vi "Framework Test.vi"() -> ()   [LabVIEW 2017]
uses:
  Source/Shared/Typedefs/DSF.Shared.Typedefs.Data Type.ctl
  Source/Shared/Typedefs/DSF.Shared.Typedefs.Direction.ctl
  Source/Shared/Typedefs/DSF.Shared.Typedefs.Cycle Timing Factors.ctl
  Source/Plugins/Reflective Memory/DSF.Transceiver.GE Reflective Memory.lvclass
  Source/Plugins/PXImc/DSF.Transceiver.PXImc.lvclass
  Source/Plugins/UDP/DSF.Transceiver.UDP.lvclass
  Source/Engine/Classes/Framework/DSF.Engine.Framework.lvclass
  <vilib>/Platform/TimedLoop/XDataNode/timing_clust.ctl
  <vilib>/Platform/TimedLoop/XDataNode/nitl_modes.ctl
  <vilib>/Platform/TimedLoop/XDataNode/wakeup.ctl
  <vilib>/National Instruments/Memory Manager/Classes/Pointer/Memory.Pointer.lvclass/Memory.Pointer.ctl
  Source/Engine/Classes/Framework/DSF.Engine.Framework.lvclass/DSF.Engine.Framework.ctl
  Source/Engine/Classes/Plugin/DSF.Engine.Plugin.lvclass/DSF.Engine.Plugin.ctl
  Source/Engine/Classes/Timing/DSF.Engine.Timing.lvclass/DSF.Engine.Timing.ctl
  <vilib>/National Instruments/Memory Manager/Classes/Pointer/Memory.Pointer.New.4B.vi
  <vilib>/National Instruments/Memory Manager/Classes/Pointer/Memory.Pointer.Write.0D.U32.vi
  <vilib>/National Instruments/Memory Manager/Classes/Pointer/Memory.Pointer.New.1B.vi
  <vilib>/National Instruments/Memory Manager/Classes/Pointer/Memory.Pointer.Write.0D.Bool.vi
  <vilib>/National Instruments/Memory Manager/Classes/Pointer/Memory.Pointer.Read.0D.Bool.vi
  <vilib>/National Instruments/Memory Manager/Classes/Pointer/Memory.Pointer.Read.0D.I32.vi
  <vilib>/National Instruments/Memory Manager/Classes/Pointer/Memory.Pointer.Read.0D.U32.vi
  <vilib>/National Instruments/Memory Manager/Classes/Pointer/Memory.Pointer.Write.0D.I32.vi
  <vilib>/National Instruments/Memory Manager/Classes/Pointer/Memory.Pointer.Allocate.vi
  <vilib>/National Instruments/Memory Manager/Classes/Pointer/Memory.Pointer.Write.No Check.0D.U32.vi
  <vilib>/National Instruments/Memory Manager/Classes/Pointer/Memory.Pointer.Parameter Check.Null Pointer.vi
  <vilib>/National Instruments/Memory Manager/Classes/Pointer/Memory.Pointer.Parameter Check.Subset.vi
  <vilib>/National Instruments/Memory Manager/Classes/Pointer/Memory.Pointer.Write.No Check.0D.Bool.vi
  <vilib>/National Instruments/Memory Manager/Classes/Pointer/Memory.Pointer.Read.No Check.0D.Bool.vi
  <vilib>/National Instruments/Memory Manager/Classes/Pointer/Memory.Pointer.Read.No Check.0D.I32.vi
  <vilib>/National Instruments/Memory Manager/Classes/Pointer/Memory.Pointer.Read.No Check.0D.U32.vi
  <vilib>/National Instruments/Memory Manager/Classes/Pointer/Memory.Pointer.Write.No Check.0D.I32.vi
  Source/Engine/Classes/Framework/DSF.Engine.Framework.Set Iteration.vi
  Source/Engine/Classes/Framework/DSF.Engine.Framework.Tx.Async.vi
  Source/Engine/Classes/Framework/DSF.Engine.Framework.Get State.vi
  Source/Engine/Classes/State/DSF.Engine.State.Framework.Get Active Plugins.vi
  Source/Engine/Classes/Framework/DSF.Engine.Framework.Get Iteration.vi
  Source/Engine/Classes/Plugin/DSF.Engine.Plugin.Iteration.Increment.vi
  Source/Engine/Classes/Plugin/DSF.Engine.Plugin.Is Active.vi
  <vilib>/National Instruments/Memory Manager/Classes/Pointer/Memory.Pointer.Set Address.vi
  <vilib>/National Instruments/Memory Manager/Classes/Pointer/Memory.Pointer.Set Size.vi
  <vilib>/National Instruments/Memory Manager/Classes/Pointer/Memory.Pointer.Set Allocated.vi
  <vilib>/National Instruments/Memory Manager/Classes/Pointer/Memory.Pointer.Get Address.vi
  <vilib>/National Instruments/Memory Manager/Classes/Pointer/Memory.Pointer.Errors.vi
  <vilib>/National Instruments/Memory Manager/Classes/Pointer/Memory.Pointer.Errors.Null Pointer.vi
  <vilib>/National Instruments/Memory Manager/Classes/Pointer/Memory.Pointer.Errors.Out of Bounds.vi
  <vilib>/National Instruments/Memory Manager/Classes/Pointer/Memory.Pointer.Get Size.vi
  Source/Engine/Classes/Plugin/DSF.Engine.Plugin.Get Timing.vi
  Source/Engine/Classes/Timing/DSF.Engine.Timing.Iteration.Increment.vi
  Source/Engine/Classes/Plugin/DSF.Engine.Plugin.Set Timing.vi
  Source/Engine/Classes/Timing/DSF.Engine.Timing.Is Active Cycle.vi
  <vilib>/National Instruments/Memory Manager/Classes/Pointer/Memory.Pointer.Errors.Create Error.vi
  <vilib>/NI/Static Error Handling/VIs/Static Error Handling.Source Buffer.Write.String.vi
  <vilib>/National Instruments/Memory Manager/Classes/Pointer/Memory.Pointer.Errors.Write Pointer Size.vi
  <vilib>/NI/Static Error Handling/VIs/Static Error Handling.Source Buffer.Write.Numeric.Scalar.Base10.vi
  <vilib>/NI/Static Error Handling/VIs/Static Error Handling.Source Buffer.Write.Numeric.Scalar.Base10 (U64).vi
  Source/Engine/Classes/Timing/DSF.Engine.Timing.Get Iteration.vi
  Source/Engine/Classes/Timing/DSF.Engine.Timing.Set Iteration.vi
  Source/Engine/Classes/Timing/DSF.Engine.Timing.Get Decimation.vi
  Source/Engine/Classes/Timing/DSF.Engine.Timing.Get Offset.vi
  <vilib>/NI/Static Error Handling/VIs/Static Error Handling.Error Cluster Constant.vi
  <vilib>/NI/Static Error Handling/VIs/Static Error Handling.Error Cluster Constant (512B).vi
  <vilib>/NI/Static Error Handling/VIs/Static Error Handling.Parameters.Status.Set.vi
  <vilib>/NI/Static Error Handling/VIs/Static Error Handling.Parameters.Code.Set.vi
  <vilib>/NI/Static Error Handling/VIs/Static Error Handling.Parameters.VI Source.Set.vi
  <vilib>/National Instruments/Memory Manager/Constants/Memory.Constants.vi
  <vilib>/National Instruments/Memory Manager/Constants/Memory.Constants.Library Name.vi
  <vilib>/National Instruments/Memory Manager/Classes/Pointer/Memory.Pointer.Errors.Get Info.vi
  Source/Engine/Classes/Plugin/DSF.Engine.Plugin.Tx.Async.vi
  <vilib>/National Instruments/Memory Manager/Classes/Pointer/Memory.Pointer.lvclass
  <vilib>/platform/TimedLoop/XDataNode/XDataNode.xnode
  <vilib>/Platform/TimedLoop/XDataNode/XDNodeRunTimeDep.lvlib
  Source/Shared/Classes/Framework/DSF.Shared.Configuration.Framework.lvclass
  Source/Engine/Classes/Pointer/DSF.Engine.Pointer.DBL.lvclass
  Source/DSF.Shared.lvlib
panel:
  out "Framework duration":u32 format="%d us"
  out "Framework Error":errorcluster
  out "Tx duration":u32 format="%d us"
  out "Rx duration":u32 format="%d us"
  out "Actual PCL Frequency":dbl format="%.0pHz"
  out "UDP Rx 2 count":i32
  out "UDP Rx 1 count":i32
  out "UDP Rx 2":errorcluster
  out "UDP Rx 1":errorcluster
  out "UDP Rx 2 port":u16
  out "UDP Rx 2 bytes":i32
  out "UDP Rx 1 bytes":i32
  out "UDP Rx 1 port":u16
  in  "Transceiver Count":i32=1
  in  "Plugins":T4(array[cluster])=[{"plugin class"="udp", "channel count per transfer"=100, "transfer configs per group"=[{"random types?"=FALSE, "non-random type"=enum."DBL"}], "group configs"=[{"direction"=enum."Tx", "timing"={"Priority"=100, "Decimation"=1, "Offset"=0}}], "plugin timing"={"Priority"=100, "Decimation"=1, "Offset"=0}}]
  in  "Configuration Path":path=path "C:/Users/Admin/Desktop/test.json"
  out "Framework Iteration":i32 format="%d cycles"
  out "Actual Period":u32 format="%d us"
  in  "Target PCL Frequency":dbl=100.0 caption="Target Period" format="%.0pHz"
  in  "stop":bool
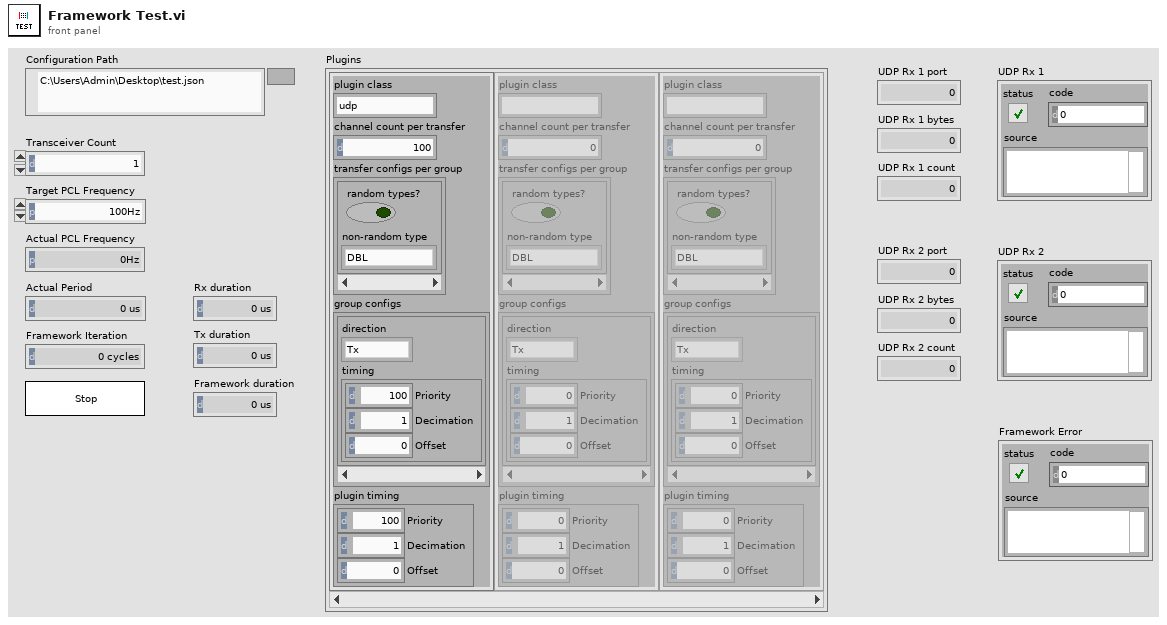
[diagram p1: front panel]
types:
  T1 = typedef "DSF.Shared.lvlib/DSF.Shared.Typedefs.Data Type.ctl" = enum8{"Bool", "SGL", "DBL", "I8", "I16", "I32", "I64", "U8", "U16", "U32", "U64"}
  T2 = typedef "DSF.Shared.lvlib/DSF.Shared.Typedefs.Direction.ctl" = enum8{"Tx", "Rx"}
  T3 = typedef "DSF.Shared.lvlib/DSF.Shared.Typedefs.Cycle Timing Factors.ctl" = cluster{"Priority":u64, "Decimation":u64, "Offset":u64}
  T4 = cluster{"plugin class":string, "channel count per transfer":i32, "transfer configs per group":cluster{"random types?":bool, "non-random type":T1}[], "group configs":cluster{"direction":T2, "timing":T3}[], "plugin timing":T3}[]
  T5 = typedef "DSF.Shared.lvlib/DSF.Shared.Refactor.Typedefs.Framework Configuration.Aggregate.ctl" = cluster{"Plugins":T6[]}
  T6 = typedef "DSF.Shared.lvlib/DSF.Shared.Refactor.Typedefs.Plugin Configuration.Aggregate.ctl" = cluster{"name":string, "class":string, "cycle timing":T3, "Transfer Groups":T7[]}
  T7 = typedef "DSF.Shared.lvlib/DSF.Shared.Refactor.Typedefs.Transfer Group Configuration.Aggregate.ctl" = cluster{"name":string, "direction":T2, "cycle timing":T3, "Transfers":T8[]}
  T8 = typedef "DSF.Shared.lvlib/DSF.Shared.Refactor.Typedefs.Transfer Configuration.ctl" = cluster{"name":string, "byte order":T9, "channel configurations":T10[]}
  T9 = typedef "DSF.Shared.lvlib/DSF.Shared.Typedefs.Byte Order.ctl" = enum8{"big-endian", "little-endian"}
  T10 = typedef "DSF.Shared.lvlib/DSF.Shared.Refactor.Typedefs.Channel Array Configuration.ctl" = cluster{"name":string, "data type":T1, "count":u64, "buffer offset":u64, "engine offset":u64}
  T11 = typedef "XDNodeRunTimeDep.lvlib/timing_clust.ctl" = cluster{"Expected End [f-1]":u64, "Actual End [f-1]":u64, "Finished Late? [f-1]":bool, "Expected End [i-1]":u64, "Actual End [i-1]":u64, "Finished Late? [i-1]":bool, "Expected Start [i]":u64, "Actual Start [i]":u64, "Expected Start [f]":u64, "Actual Start [f]":u64, "Source Name":string, "Structure Name":string, "Period":i64, "Deadline":i64, "Offset":i64, "Start":i64, "Priority":i32, "Timeout":i32, "Mode":T12, "Wakeup Reason":T13, "Error":errorcluster, "Source Type":string, "Secondary Source Type":string, "Global End Time":u64, "Global Start Time":u64, "Frame Duration":u64, "Iteration Duration":u64, "Assigned CPU":i32, "I/O Scan Engine Mode":u32}
  T12 = typedef "XDNodeRunTimeDep.lvlib/nitl_modes.ctl" = enum32{"No Change", "Process missed periods, maintain original phase", "Discard missed periods, maintain original phase", "Process missed periods, ignore original phase", "Discard missed periods, ignore original phase"}
  T13 = typedef "XDNodeRunTimeDep.lvlib/wakeup.ctl" = enum32{"Normal", "Aborted", "Asynchronous wakeup", "Timing source error", "Timed loop error", "Timeout"}
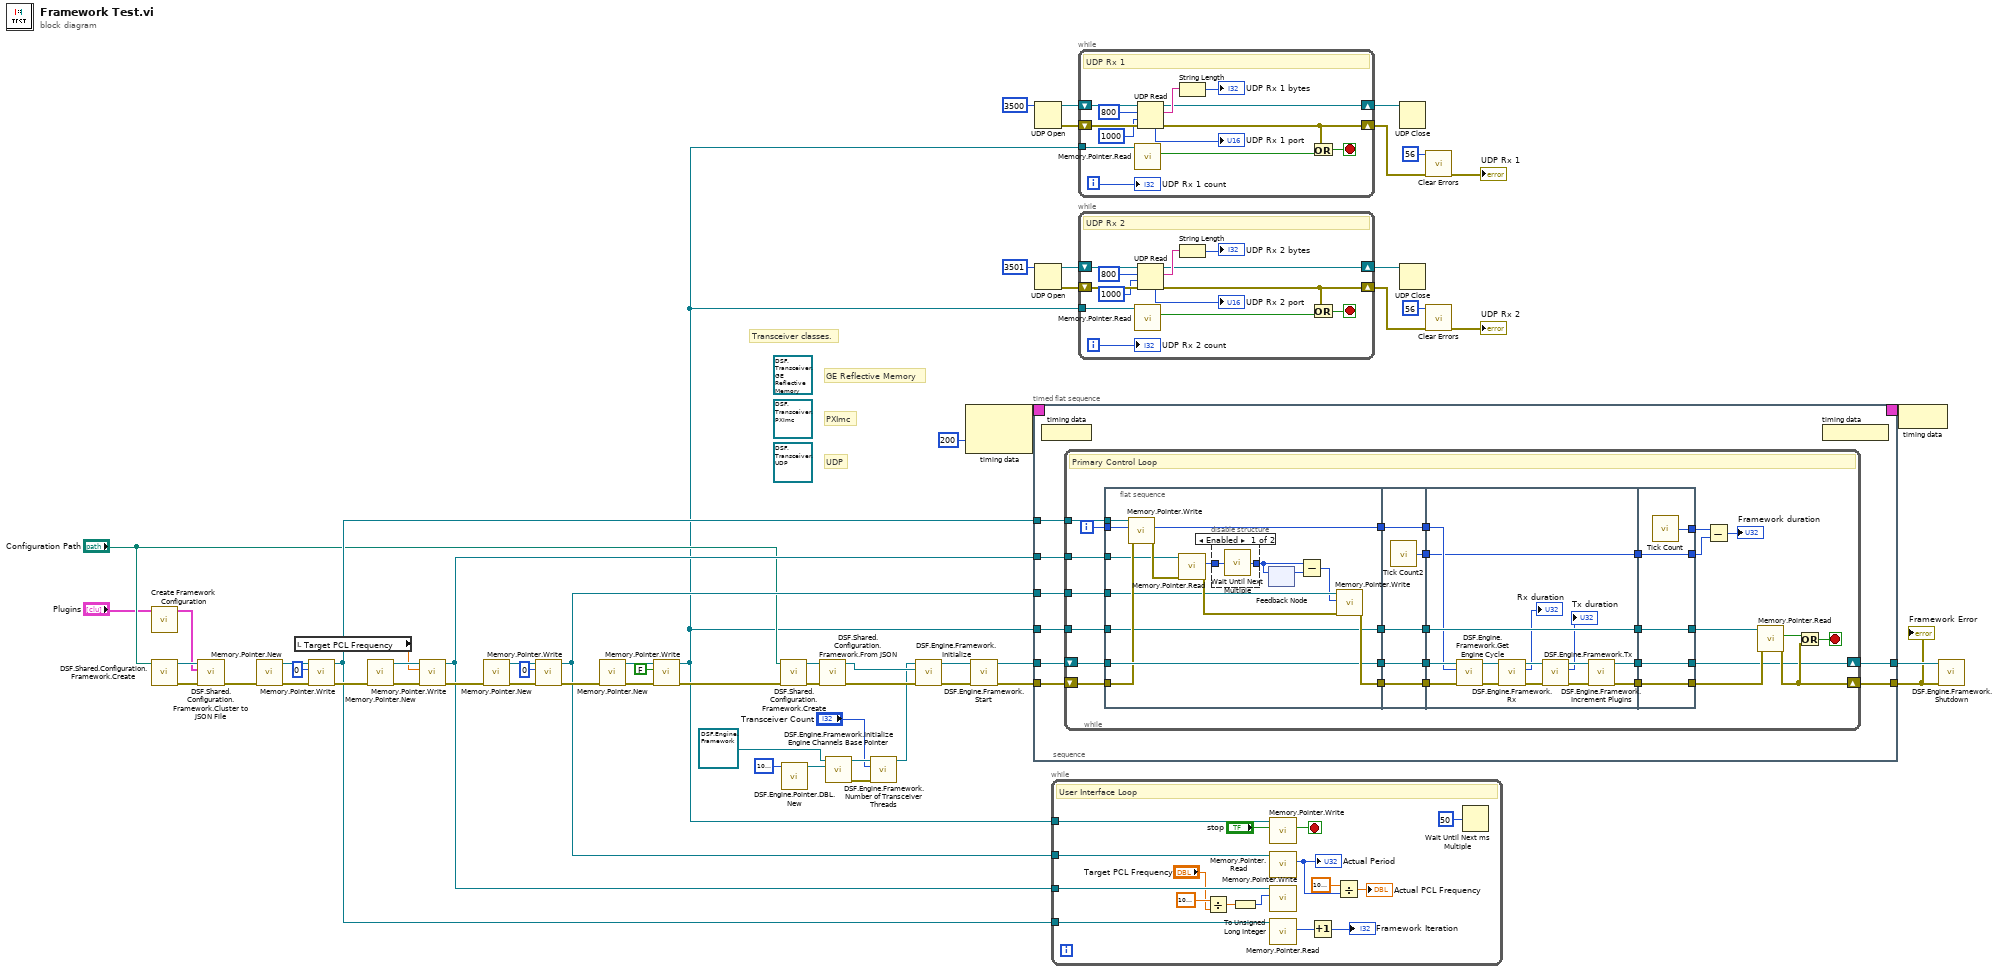
[diagram p0: block diagram]
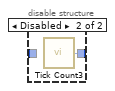
[diagram p2: hidden frame]
diagram:
  (unwired) refnum<class "DSF.Transceiver.UDP.lvclass"> refnum ("DSF UDP Transceiver")
  (unwired) refnum<class "DSF.Transceiver.PXImc.lvclass"> refnum ("DSF PXImc Transceiver")
  (unwired) refnum<class "DSF.Transceiver.GE Reflective Memory.lvclass"> refnum ("DSF GE Reflective Memory Transceiver")
  # "Transceiver classes."
  # "UDP"
  # "PXImc"
  # "GE Reflective Memory"
  n1 = call "Create Framework Configuration.vi"("Plugins"="Plugins") -> ("Framework Configuration"=w28:T5)  [unwired: 10 in]
  n2 = call "DSF.Shared.Configuration.Framework.Create.vi"("configuration path"="Configuration Path") -> ("error out"=w29:errorcluster, "Framework Configuration"=w30:refnum<class "DSF.Shared.Configuration.Framework.lvclass">)  [unwired: 9 in]
  n3 = call "DSF.Shared.Configuration.Framework.Cluster to JSON File.vi"("error in (no error)"=w29, "Framework Configuration"=w28, "Framework Configuration in"=w30) -> ("error out"=w27:errorcluster)  [unwired: 7 in, 1 out]
  n4 = call-poly <vilib>:"Memory.Pointer.New.vi"("error in (no error)"=w27) -> ("error out"=w37:errorcluster, "Pointer"=w39:refnum<class "Memory.Pointer.lvclass">)  [unwired: 9 in]
  n5 = local read "Target PCL Frequency"() -> (w47:dbl)
  n6 = call-poly <vilib>:"Memory.Pointer.Write.vi"("error in (no error)"=w37, "value"=u32 0, "Pointer in"=w39) -> ("error out"=w36:errorcluster, "Pointer out"=w33:refnum<class "Memory.Pointer.lvclass">)  [unwired: 5 in, 2 out]
  n7 = call-poly <vilib>:"Memory.Pointer.New.vi"("error in (no error)"=w36) -> ("error out"=w46:errorcluster, "Pointer"=w48:refnum<class "Memory.Pointer.lvclass">)  [unwired: 9 in]
  n8 = call-poly <vilib>:"Memory.Pointer.Write.vi"("error in (no error)"=w46, "value"=w47, "Pointer in"=w48) -> ("error out"=w45:errorcluster, "Pointer out"=w40:refnum<class "Memory.Pointer.lvclass">)  [unwired: 5 in, 2 out]
  n9 = call-poly <vilib>:"Memory.Pointer.New.vi"("error in (no error)"=w45) -> ("error out"=w43:errorcluster, "Pointer"=w49:refnum<class "Memory.Pointer.lvclass">)  [unwired: 9 in]
  n10 = call-poly <vilib>:"Memory.Pointer.Write.vi"("error in (no error)"=w43, "value"=u32 0, "Pointer in"=w49) -> ("error out"=w42:errorcluster, "Pointer out"=w41:refnum<class "Memory.Pointer.lvclass">)  [unwired: 5 in, 2 out]
  n11 = call-poly <vilib>:"Memory.Pointer.New.vi"("error in (no error)"=w42) -> ("error out"=w52:errorcluster, "Pointer"=w51:refnum<class "Memory.Pointer.lvclass">)  [unwired: 9 in]
  n12 = call-poly <vilib>:"Memory.Pointer.Write.vi"("error in (no error)"=w52, "value"=FALSE, "Pointer in"=w51) -> ("error out"=w31:errorcluster, "Pointer out"=w17:refnum<class "Memory.Pointer.lvclass">)  [unwired: 5 in, 2 out]
  n13 = call "DSF.Shared.Configuration.Framework.Create.vi"("error in (no error)"=w31, "configuration path"="Configuration Path") -> ("error out"=w34:errorcluster, "Framework Configuration"=w35:refnum<class "DSF.Shared.Configuration.Framework.lvclass">)  [unwired: 8 in]
  n14 = call "DSF.Engine.Pointer.DBL.New.vi"("channel count"=u64 1000000) -> ("DBL Pointer out"=w23:refnum<class "DSF.Engine.Pointer.DBL.lvclass">)  [unwired: 9 in, 1 out]
  n15 = call "DSF.Shared.Configuration.Framework.From JSON.vi"("error in (no error)"=w34, "Framework Configuration in"=w35) -> ("error out"=w60:errorcluster, "Framework Configuration out"=w24:refnum<class "DSF.Shared.Configuration.Framework.lvclass">)  [unwired: 8 in]
  n16 = call-dynamic "DSF.Engine.Framework.Initialize Engine Channels Base Pointer.vi"("Engine Channels Pointer"=w23, "Framework in"=refnum<class "DSF.Engine.Framework.lvclass"> refnum) -> ("error out"=w15:errorcluster, "Framework out"=w20:refnum<class "DSF.Engine.Framework.lvclass">)  [unwired: 8 in]
  n17 = call "DSF.Engine.Framework.Number of Transceiver Threads.vi"("error in (no error)"=w15, "transceiver count"="Transceiver Count", "Framework in"=w20) -> ("Framework out"=w19:refnum<class "DSF.Engine.Framework.lvclass">)  [unwired: 7 in, 1 out]
  n18 = call "DSF.Engine.Framework.Initialize.vi"("error in (no error)"=w60, "Framework Configuration"=w24, "Framework type"=w19) -> ("error out"=w59:errorcluster, "Framework out"=w32:refnum<class "DSF.Engine.Framework.lvclass">)  [unwired: 7 in]
  n19 = node-c288(200 ("Priority")) -> (w54:T11)  [unwired: 1 in]
  n20 = call "DSF.Engine.Framework.Start.vi"("error in (no error)"=w59, "Framework in"=w32) -> ("error out"=w57:errorcluster, "Framework out"=w58:refnum<class "DSF.Engine.Framework.lvclass">)  [unwired: 8 in]
  n21 = timed-sequence {
    timing: w54 -> [_]
    timing-out: [_] -> w53
    tunnel: w58 -> [w68]
    tunnel: w57 -> [w67]
    tunnel: [w66] -> w56
    tunnel: [w65] -> w55
    tunnel: w17 -> [w64]
    tunnel: w40 -> [w63]
    tunnel: w41 -> [w62]
    tunnel: w33 -> [w61]
    n22 = timed-flat-sequence {
      tunnel: w68 -> [w76]
      tunnel: w67 -> [w75]
      tunnel: [w74] -> w66
      tunnel: [w73] -> w65
      tunnel: w64 -> [w72]
      tunnel: w63 -> [w71]
      tunnel: w62 -> [w70]
      tunnel: w61 -> [w69]
      n23 = node-c288() -> ()  [unwired: 1 in]
      n24 = while {
        shift-right: [w95] -> w74
        shift-left: w76 -> [w104]
        shift-right: [w97] -> w73
        shift-left: w75 -> [w105]
        tunnel: w72 -> [w103]
        tunnel: w71 -> [w101]
        tunnel: w70 -> [w100]
        tunnel: w69 -> [w94]
        i -> [w93]
        stop <- w96 stop-if-true
        # "Primary Control Loop"
        n25 = flat-sequence {
          tunnel: w105 -> [w113]
          tunnel: w104 -> [w118]
          tunnel: w103 -> [w109]
          tunnel: [w119] -> w85
          tunnel: [w118] -> w83
          tunnel: [w109] -> w81
          tunnel: w101 -> [w111]
          tunnel: w100 -> [w110]
          tunnel: w94 -> [w115]
          tunnel: w93 -> [w114]
          tunnel: [w108] -> w79
          tunnel: w85 -> [w128]
          tunnel: [w128] -> w84
          tunnel: w83 -> [w127]
          tunnel: [w127] -> w82
          tunnel: w81 -> [w126]
          tunnel: [w126] -> w80
          tunnel: w79 -> [w125]
          tunnel: [w125] -> w78
          tunnel: [w124] -> w77
          tunnel: w84 -> [w139]
          tunnel: w82 -> [w140]
          tunnel: w80 -> [w143]
          tunnel: w78 -> [w138]
          tunnel: w77 -> [w129]
          tunnel: [w143] -> w92
          tunnel: [w135] -> w91
          tunnel: [w134] -> w90
          tunnel: [w129] -> w89
          tunnel: [w146] -> w99
          tunnel: [w147] -> w95
          tunnel: [w148] -> w102
          tunnel: w92 -> [w148]
          tunnel: w91 -> [w147]
          tunnel: w90 -> [w146]
          tunnel: [w145] -> w88
          tunnel: w89 -> [w144]
          tunnel: [w144] -> w87
          frame #0 {
            n26 = call-poly <vilib>:"Memory.Pointer.Write.vi"("error in (no error)"=w113, "value"=w114, "Pointer in"=w115) -> ("error out"=w112:errorcluster, "value"=w108:i32)  [unwired: 5 in, 2 out]
            n27 = call-poly <vilib>:"Memory.Pointer.Read.vi"("error in (no error)"=w112, "Pointer in"=w111) -> ("error out"=w116:errorcluster, "value out"=w117:u32)  [unwired: 6 in, 2 out]
            n28 = disable-structure shown="Enabled" {
              disable-tunnel: w117 -> [w122 _]
              disable-tunnel: [w121 w123] -> w106
              frame Enabled {
                n29 = call "Wait Until Next Multiple"("Count(uSec)"=w122) -> ("Tick Count(uSec)"=w121:u32)
              }
              frame Disabled {
                n30 = call "Tick Count3"() -> ("Tick Count(uSec)"=w123:u32)
              }
            }
            n31 = feedback #1() -> (w120:u32)  [unwired: 1 in]
            n32 = feedback-in #1(w106) -> ()
            n33 = Subtract(x=w106, y=w120) -> (x-y=w107:u32)
            n34 = call-poly <vilib>:"Memory.Pointer.Write.vi"("error in (no error)"=w116, "value"=w107, "Pointer in"=w110) -> ("error out"=w119:errorcluster)  [unwired: 5 in, 3 out]
          }
          frame #1 {
            n35 = call "Tick Count2"() -> ("Tick Count(uSec)"=w124:u32)
          }
          frame #2 {
            n36 = call "DSF.Engine.Framework.Get Engine Cycle.vi"("error in (no error)"=w139, "iteration"=w138, "Framework in"=w140) -> ("error out"=w130:errorcluster, "Framework out"=w131:refnum<class "DSF.Engine.Framework.lvclass">)  [unwired: 7 in]
            n37 = call "DSF.Engine.Framework.Rx.vi"("error in (no error)"=w130, "Framework in"=w131) -> ("error out"=w142:errorcluster, "duration"=→"Rx duration":u32, "Framework out"=w141:refnum<class "DSF.Engine.Framework.lvclass">)  [unwired: 7 in]
            n38 = call "DSF.Engine.Framework.Tx.vi"("error in (no error)"=w142, "Framework in"=w141) -> ("error out"=w136:errorcluster, "duration"=→"Tx duration":u32, "Framework out"=w137:refnum<class "DSF.Engine.Framework.lvclass">)  [unwired: 7 in]
            n39 = call "DSF.Engine.Framework.Increment Plugins.vi"("error in (no error)"=w136, "Framework in"=w137) -> ("error out"=w134:errorcluster, "Framework out"=w135:refnum<class "DSF.Engine.Framework.lvclass">)  [unwired: 8 in]
          }
          frame #3 {
            n40 = call "Tick Count"() -> ("Tick Count(uSec)"=w145:u32)
          }
        }
        n41 = Subtract(x=w88, y=w87) -> (x-y=→"Framework duration":u32)
        n42 = call-poly <vilib>:"Memory.Pointer.Read.vi"("error in (no error)"=w99, "Pointer in"=w102) -> ("error out"=w97:errorcluster, "value out"=w98:bool)  [unwired: 6 in, 2 out]
        n43 = Or(x=w98, y=w97) -> (x .or. y?=w96:bool)
      }
      n44 = node-c288() -> ()  [unwired: 1 out]
    }
  }
  "Framework Error" <- w55
  n45 = UDP Open(11:u16 3500 ("port")) -> (port=w14:refnum<k16>, 0:w13:errorcluster)  [unwired: 4 in, 1 out]
  n46 = UDP Open(11:u16 3501 ("port")) -> (port=w9:refnum<k16>, 0:w10:errorcluster)  [unwired: 4 in, 1 out]
  n47 = while {
    tunnel: w17 -> [w165]
    tunnel: w41 -> [w160]
    tunnel: w40 -> [w161]
    tunnel: w33 -> [w152]
    stop <- w166 stop-if-true
    # "User Interface Loop"
    n48 = Divide(x=1000000.0 ("y"), y="Target PCL Frequency") -> (x/y=w156:dbl)
    n49 = To Unsigned Long Integer(number=w156) -> (unsigned 32bit integer=w154:u32)
    n50 = call-poly <vilib>:"Memory.Pointer.Write.vi"("value"="stop", "Pointer in"=w165) -> ("value"=w166:bool)  [unwired: 6 in, 3 out]
    n51 = call-poly <vilib>:"Memory.Pointer.Read.vi"("Pointer in"=w160) -> ("value out"=w157:u32)  [unwired: 7 in, 3 out]
    "Actual Period" <- w157
    n52 = call-poly <vilib>:"Memory.Pointer.Write.vi"("value"=w154, "Pointer in"=w161) -> ()  [unwired: 6 in, 4 out]
    n53 = call-poly <vilib>:"Memory.Pointer.Read.vi"("Pointer in"=w152) -> ("value out"=w162:i32)  [unwired: 7 in, 3 out]
    n54 = Increment(x=w162) -> (x+1=→"Framework Iteration":i32)
    n55 = Divide(x=1000000.0, y=w157) -> (x/y=→"Actual PCL Frequency":dbl)
    n56 = Wait Until Next ms Multiple(millisecond multiple=u32 50 ("milliseconds to wait")) -> ()  [unwired: 1 out]
  }
  n57 = while {
    shift-right: [w170] -> w5
    shift-left: w13 -> [w178]
    shift-right: [w175] -> w8
    shift-left: w14 -> [w179]
    tunnel: w17 -> [w173]
    i -> [w168]
    stop <- w171 stop-if-true
    # "UDP Rx 1"
    n58 = call-poly <vilib>:"Memory.Pointer.Read.vi"("Pointer in"=w173) -> ("value out"=w172:bool)  [unwired: 7 in, 3 out]
    n59 = UDP Read(connection ID=w179, max size (548)=800, timeout ms (25000)=1000, 8:w178) -> (data out=w177:string, error out=w170:errorcluster, 3:w175:refnum<k16>, 4:→"UDP Rx 1 port":u16)  [unwired: 1 out]
    n60 = String Length(string=w177) -> (length=→"UDP Rx 1 bytes":i32)
    n61 = Or(x=w170, y=w172) -> (x .or. y?=w171:bool)
    "UDP Rx 1 count" <- w168
  }
  n62 = while {
    shift-right: [w183] -> w2
    shift-left: w10 -> [w191]
    shift-right: [w188] -> w7
    shift-left: w9 -> [w192]
    tunnel: w17 -> [w186]
    i -> [w181]
    stop <- w184 stop-if-true
    # "UDP Rx 2"
    n63 = call-poly <vilib>:"Memory.Pointer.Read.vi"("Pointer in"=w186) -> ("value out"=w185:bool)  [unwired: 7 in, 3 out]
    n64 = UDP Read(connection ID=w192, max size (548)=800, timeout ms (25000)=1000, 8:w191) -> (data out=w190:string, error out=w183:errorcluster, 3:w188:refnum<k16>, 4:→"UDP Rx 2 port":u16)  [unwired: 1 out]
    n65 = String Length(string=w190) -> (length=→"UDP Rx 2 bytes":i32)
    n66 = Or(x=w183, y=w185) -> (x .or. y?=w184:bool)
    "UDP Rx 2 count" <- w181
  }
  n67 = UDP Close(connection ID=w8) -> ()  [unwired: 1 in, 2 out]
  n68 = UDP Close(connection ID=w7) -> ()  [unwired: 1 in, 2 out]
  n69 = call <vilib>:"Clear Errors.vi"("error in (no error)"=w5, "specific error code to clear (0: all)"=56) -> ("error out"=→"UDP Rx 1":errorcluster)  [unwired: 4 in, 1 out]
  n70 = call <vilib>:"Clear Errors.vi"("error in (no error)"=w2, "specific error code to clear (0: all)"=56) -> ("error out"=→"UDP Rx 2":errorcluster)  [unwired: 4 in, 1 out]
  n71 = node-c288(w53) -> ()
  n72 = call "DSF.Engine.Framework.Shutdown.vi"("error in (no error)"=w55, "Framework in"=w56) -> ()  [unwired: 8 in, 2 out]
